vi "NewBackground.vi"(8 "error in (no error)":errorcluster, 11 "Snake in":refnum<class "SnakeGame.lvclass">) -> (0 "error out":errorcluster, 3 "Snake out":refnum<class "SnakeGame.lvclass">)   [LabVIEW 2019, in "RT_Game.lvlib" / "SnakeGame.lvclass"]
uses:
  SnakeGame.lvclass
  SnakeGame.lvclass/SnakeGame.ctl
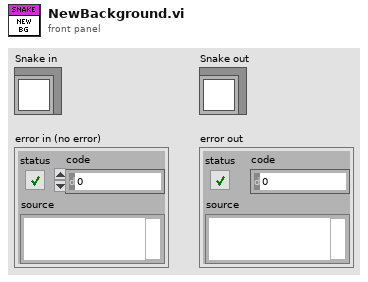
[diagram p1: front panel]
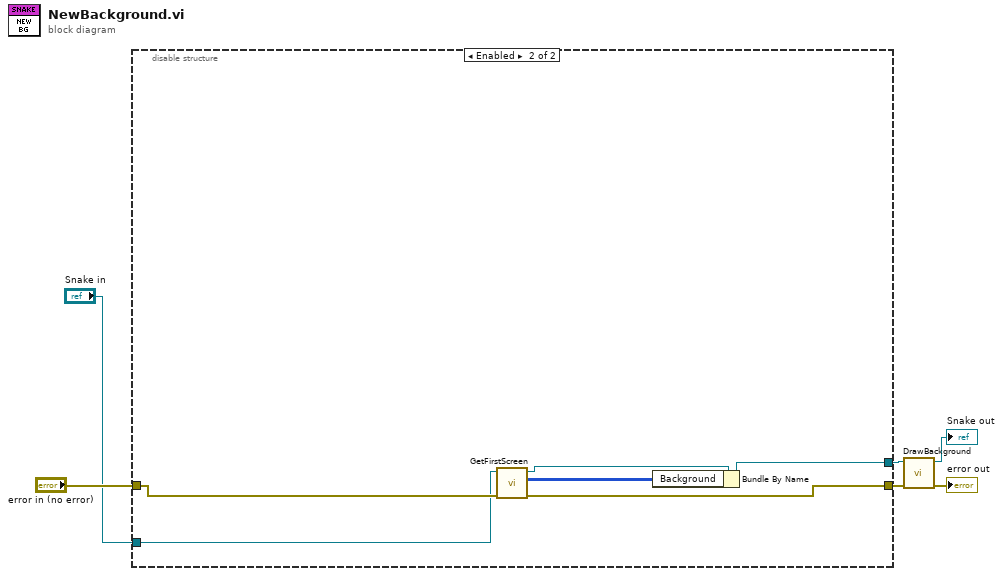
[diagram p0: block diagram]
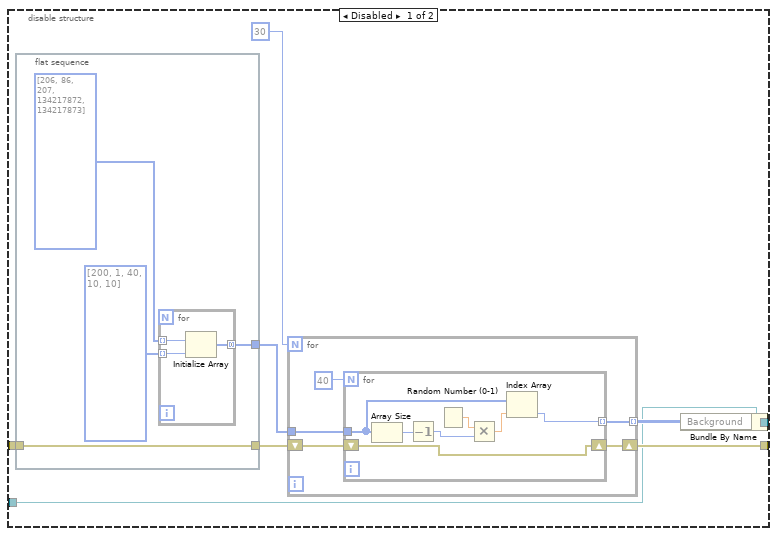
[diagram p2: hidden frame]
diagram:
  n1 = disable-structure shown="Enabled" {
    disable-tunnel: [w12 w38] -> w6
    disable-tunnel: [w11 w37] -> w3
    disable-tunnel: "error in (no error)" -> [w9 w39]
    disable-tunnel: "Snake in" -> [w7 w36]
    frame Disabled {
      n2 = flat-sequence {
        tunnel: [w16] -> w10
        tunnel: [w15] -> w8
        tunnel: w9 -> [w15]
        frame #0 {
          n3 = for {
            tunnel: u32[] [206, 86, 207, 134217872, 134217873] -> [w20] mode=indexing
            tunnel: i32[] [200, 1, 40, 10, 10] -> [w21] mode=indexing
            tunnel: [w19] -> w16 mode=concatenating
            n4 = Initialize Array(w20, w21) -> (w19:u32[])
          }
        }
      }
      n5 = for {
        N: 30 -> [_]
        tunnel: [w26] -> w14 mode=indexing
        shift-right: [w24] -> w11
        shift-left: w8 -> [w23]
        tunnel: w10 -> [w22]
        n6 = for {
          N: 40 -> [_]
          tunnel: [w27] -> w26 mode=indexing
          shift-right: [w28] -> w24
          shift-left: w23 -> [w28]
          tunnel: w22 -> [w29]
          n7 = Array Size(array=w29) -> (size(s)=w31:i32)
          n8 = Decrement(x=w31) -> (x-1=w30:i32)
          n9 = Random Number (0-1)() -> (number: 0 to 1=w33:dbl)
          n10 = Multiply(x=w33, y=w30) -> (x*y=w32:dbl)
          n11 = Index Array(array=w29, index=w32) -> (element=w27:u32)
        }
      }
      n12 = Bundle By Name(cluster=w7, "Background"=w14) -> (w12:refnum<class "SnakeGame.lvclass">)
    }
    frame Enabled {
      n13 = call-dynamic "GetFirstScreen.vi"("error in (no error)"=w39, "SnakeGame in"=w36) -> ("error out"=w37:errorcluster, "Array"=w34:u32[][], "SnakeGame out"=w35:refnum<class "SnakeGame.lvclass">)  [unwired: 7 in]
      n14 = Bundle By Name(cluster=w35, "Background"=w34) -> (w38:refnum<class "SnakeGame.lvclass">)
    }
  }
  n15 = call "DrawBackground.vi"("error in (no error)"=w3, "Snake in"=w6) -> ("error out"=→"error out":errorcluster, "Snake out"=→"Snake out":refnum<class "SnakeGame.lvclass">)  [unwired: 8 in]
